vi "Process.vi"(8 "error in (no error)":errorcluster, 11 "Spectral Processing in":refnum<class "Spectral Processing.lvclass">) -> (0 "error out":errorcluster, 3 "Spectral Processing out":refnum<class "Spectral Processing.lvclass">)   [LabVIEW 2014, in "Spectral Processing.lvclass"]
uses:
  Spectral Processing.lvclass
panel:
  in  "A-Scan":u16[](array[numeric])
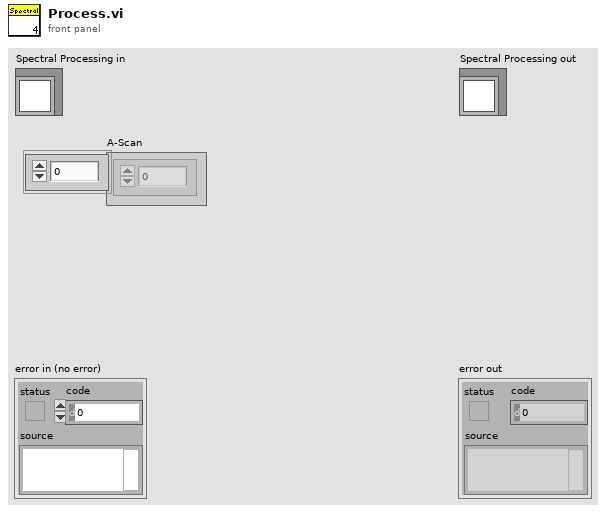
[diagram p1: front panel]
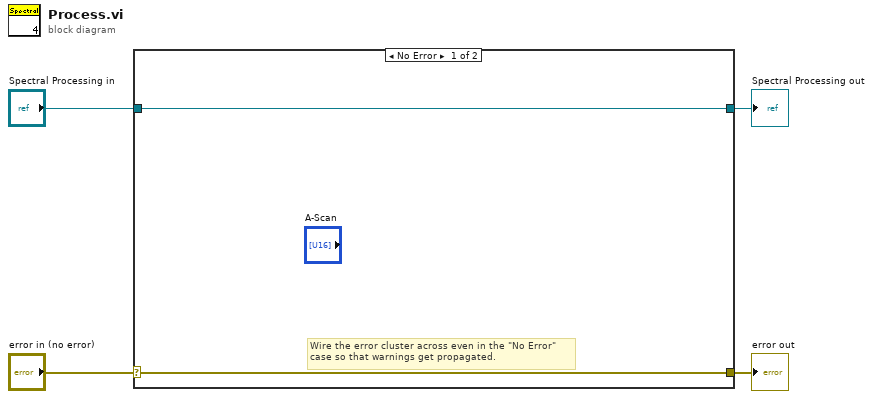
[diagram p0: block diagram]
diagram:
  n1 = case shown="No Error" "error in (no error)" {
    selector: "error in (no error)" -> [w5 w8]
    tunnel: [w5 w8] -> w3
    tunnel: [w6 w7] -> w1
    tunnel: "Spectral Processing in" -> [w6 w7]
    frame No Error {
      # "Wire the error cluster across even in the \"No Error\"\ncase so that warnings get propagated."
    }
    frame Error {
    }
  }
  "error out" <- w3
  "Spectral Processing out" <- w1
